vi "Command Handler.vi"   [LabVIEW 2017, in "HD44780 FPGA.lvlib"]
doc: "Receives and parses commands from the Host VIs or FPGA VIs."
uses:
  HD44780 FPGA.lvlib
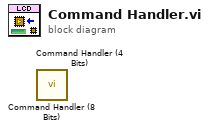
[diagram p0: block diagram]
diagram:
  n1 = call "Command Handler (8 Bits).vi"() -> ()  [unwired: 11 in, 1 out]
  n2 = call "Command Handler (4 Bits).vi"() -> ()  [unwired: 11 in, 1 out]
